vi "reward_behavior_michelle_visjitter_conswinAdapt_enticefx_TSLog_VF_withvid.vi"() -> ()   [LabVIEW 2019]
doc: "The myRIO Project template acquires acceleration data from the onboard accelerometer and displays the changes of acceleration values in a waveform chart."
uses:
  <vilib>/Analysis/Matrix/Datatypes/RealMatrix.ctl
  <vilib>/myRIO/Instrument Drivers/Onboard IO/DIO/typedefs/DIO Reference.ctl
  <vilib>/myRIO/Common/Instrument Driver Framework/Utilities/typedefs/myRIO Generic Hardware Reference.ctl
  <vilib>/myRIO/Common/Instrument Driver Framework/Utilities/typedefs/Hardware Version Enum.ctl
  <vilib>/myRIO/Common/Instrument Driver Framework/Utilities/typedefs/myRIO v1.0 Reference.ctl
  <vilib>/myRIO/Common/Instrument Driver Framework/Utilities/typedefs/Generic FPGA Reference.ctl
  <vilib>/myRIO/Common/Instrument Driver Framework/myRIO v1.0/DIO/typedefs/DIO Channels List.ctl
  <vilib>/myRIO/Common/Instrument Driver Framework/myRIO v1.0/DIO/typedefs/DIO Channels Enum.ctl
  <vilib>/userdefined/High Color/nirio_resource_hc.ctl
  <vilib>/myRIO/Common/Instrument Driver Framework/myRIO v1.0/Encoder/typedefs/Encoder Signal Mode.ctl
  <vilib>/myRIO/Instrument Drivers/Onboard IO/Encoder/typedefs/Encoder Reference.ctl
  <vilib>/myRIO/Common/Instrument Driver Framework/myRIO v1.0/Encoder/typedefs/Encoder Channels Enum.ctl
  <vilib>/myRIO/Common/Instrument Driver Framework/myRIO v1.0/Encoder/typedefs/Encoder Configuration v1.0.ctl
  <vilib>/myRIO/Common/Instrument Driver Framework/Utilities/vis/Is FPGA Ref Available.vi
  <vilib>/myRIO/Common/Instrument Driver Framework/myRIO v1.0/DIO/vis/myRIO v1.1 Open DIO.vi
  <vilib>/myRIO/Instrument Drivers/Onboard IO/DIO/vis/Write.vi
  <vilib>/myRIO/Common/Instrument Driver Framework/myRIO v1.0/Encoder/vis/myRIO v1.1 Open Encoder.vi
  <vilib>/myRIO/Instrument Drivers/Onboard IO/Encoder/vis/Read.vi
  <vilib>/myRIO/Instrument Drivers/Onboard IO/DIO/vis/Read.vi
  <vilib>/myRIO/Common/Instrument Driver Framework/Utilities/vis/Validate Channels.vi
  <vilib>/myRIO/Common/Instrument Driver Framework/myRIO v1.0/DIO/vis/myRIO v1.0 Reserve DIO.vi
  <vilib>/myRIO/Common/Instrument Driver Framework/myRIO v1.0/Encoder/vis/myRIO v1.0 Reserve Encoder.vi
  <vilib>/myRIO/Common/Instrument Driver Framework/myRIO v1.0/Resource Manager/vis/myRIO v1.0 Reserve Channel List.vi
  <vilib>/myRIO/Common/Instrument Driver Framework/myRIO v1.0/DIO/vis/myRIO v1.0 Build MUX Configuration DIO.vi
  <vilib>/myRIO/Common/Instrument Driver Framework/myRIO v1.0/Encoder/vis/myRIO v1.0 Build MUX Configuration Encoder.vi
  <vilib>/myRIO/Common/Instrument Driver Framework/myRIO v1.0/Resource Manager/vis/myRIO v1.0 Reserve Channel.vi
  <vilib>/myRIO/Common/Instrument Driver Framework/myRIO v1.0/Resource Manager/vis/myRIO v1.0 Unreserve Channel.vi
  <vilib>/myRIO/Common/Instrument Driver Framework/myRIO v1.0/Resource Manager/vis/myRIO v1.0 Create Configuration List.vi
  <vilib>/myRIO/Common/Instrument Driver Framework/myRIO v1.0/Resource Manager/vis/myRIO v1.0 Build Mutex Name.vi
  <vilib>/Utility/VariantDataType/GetNumericInfo.vi
  <vilib>/Utility/error.llb/Error Cluster From Error Code.vi
  <vilib>/myRIO/Common/Instrument Driver Framework/myRIO v1.0/myRIO v1.1 Open.vi
  <vilib>/myRIO/Common/Instrument Driver Framework/Utilities/vis/IO Manager.vi
  <vilib>/myRIO/Common/Instrument Driver Framework/Utilities/vis/Configuration Manager.vi
  <vilib>/myRIO/Common/Instrument Driver Framework/myRIO v1.0/Resource Manager/vis/myRIO v1.0 Configure IO.vi
  <vilib>/myRIO/Common/Instrument Driver Framework/myRIO v1.0/myRIO v1.0 Close.vi
  <vilib>/myRIO/Common/Instrument Driver Framework/myRIO v1.0/Encoder/vis/myRIO v1.0 Configure Encoder.vi
  <vilib>/myRIO/Common/Instrument Driver Framework/myRIO v1.0/Encoder/vis/myRIO v1.0 Read Encoder.vi
  <vilib>/myRIO/Common/Instrument Driver Framework/myRIO v1.0/DIO/vis/myRIO v1.0 Write DIO.vi
  <vilib>/myRIO/Common/Instrument Driver Framework/myRIO v1.0/DIO/vis/myRIO v1.0 Read DIO.vi
  <vilib>/myRIO/Express VI/Onboard IO/Encoder/Encoder Express VI.xnode
  <vilib>/myRIO/Instrument Drivers/Onboard IO/Encoder/vis/myRIO Encoder Open.xnode
  <vilib>/myRIO/Common/Instrument Driver Framework/myRIO v1.0/Encoder/typedefs/Encoder Count Direction Enum.ctl
  <vilib>/myRIO/Express VI/Onboard IO/DO/DO Express VI.xnode
  <vilib>/myRIO/Instrument Drivers/Onboard IO/DIO/vis/myRIO DIO Open.xnode
  <vilib>/myRIO/Express VI/Onboard IO/DI/DI Express VI.xnode
  <vilib>/myRIO/Instrument Drivers/Onboard IO/Encoder/Encoder.lvlib
  <vilib>/myRIO/Instrument Drivers/Onboard IO/DIO/DIO.lvlib
  <vilib>/Analysis/Matrix/NI_Matrix.lvlib
panel:
  out "GetVidFrame":i32
  out "VidTS":dbl[][](array[numeric])
  out "VidFrameClock":i32
  out "EntTS":dbl[][](array[numeric])
  out "TimeLag":dbl
  out "Lag2":dbl
  out "TestTime":dbl
  out "RewTS":dbl[][](array[numeric])
  out "ConsTS":dbl[][](array[numeric])
  out "LickTS":dbl[][](array[numeric])
  out "ContrastChoice":dbl
  out "Its":i32
  out "BurstCriteria":dbl
  out "LickBurst 2":bool
  out "LickBurst":bool
  out "Enticements":i32
  in  "Entice":bool
  out "Misses":i32
  out "GoAhead":bool
  out "TimeOutDuration":i32
  out "ActiveTime":dbl
  out "ConsumptionGo":bool=TRUE
  out "Consumption_Period":i32
  out "Watch_Display":bool=TRUE
  in  "Give reward":bool
  out "Timings":dbl[](array[numeric])
  out "ISI":dbl
  out "ISI start time":dbl
  out "Time_out":bool=TRUE
  out "Time since lick":dbl
  out "Time of last lick":dbl
  out "Rewarded trials":dbl[](array[numeric])
  out "Rewards":u16
  out "Active Trial":bool
  out "Array temp2":T1
  out "Stimuli Loaded":bool
  out "Stim_ID":dbl[](array[numeric])
  out "Reward_mat":dbl[](array[numeric])
  out "Reward":bool=TRUE
  out "Frame clock":i32
  out "Licks":u32
  out "Lick":bool
  out "Time":dbl
  out "Stop":bool
  in  "Frames to collect":u32
  out "Overflow?":bool
  out "Counter Value":i32
  out "Velocity":dbl
  out "Velocity Plot":dbl[](graph)
  out "Velocity array":dbl[](array[numeric])
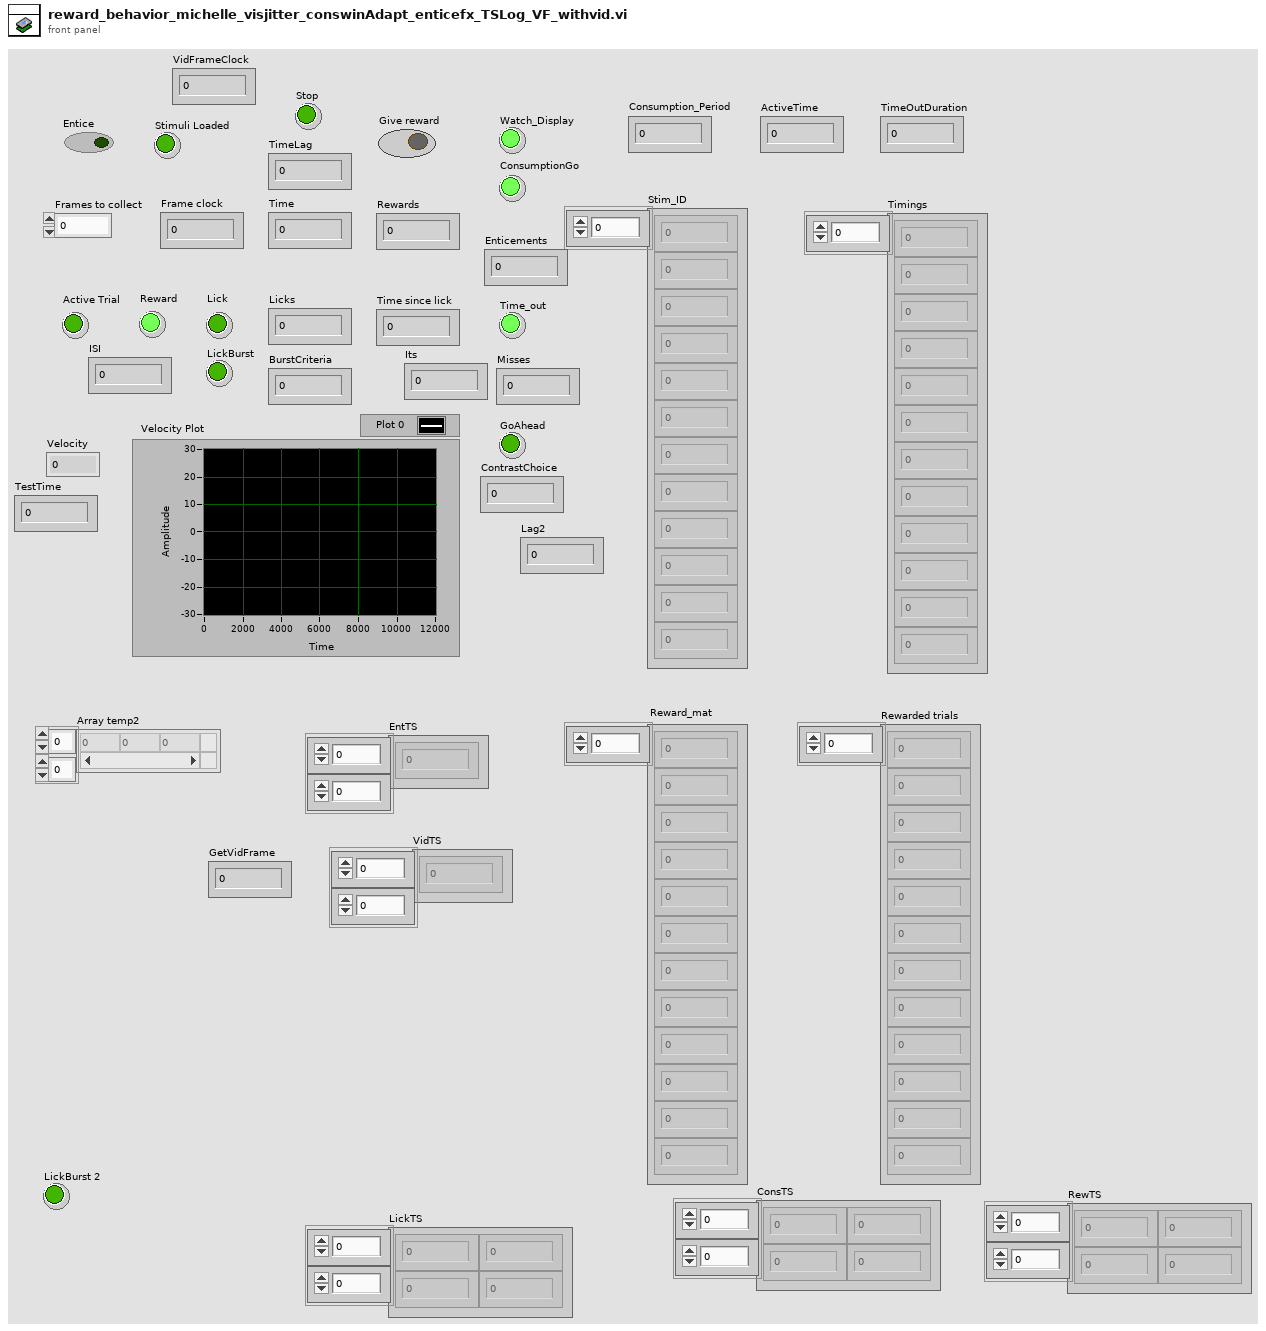
[diagram p1: front panel]
types:
  T1 = typedef "NI_Matrix.lvlib/RealMatrix.ctl" = dbl[][]
  T2 = typedef "DIO.lvlib/DIO Reference.ctl" = cluster{"myRIO Reference":T3, "DIO Channels List":T7}
  T3 = typedef "myRIO Generic Hardware Reference.ctl" = cluster{"myRIO Model":T4, "myRIO Hardware Reference":T5}
  T4 = typedef "Hardware Version Enum.ctl" = enum16{"Unknown", "myRIO-1900", "myRIO-1950", "roboRIO", "NI ELVIS RIO CM", "ELVIS III"}
  T5 = typedef "myRIO v1.0 Reference.ctl" = cluster{"Generic FPGA Reference":T6, "Allow multiple opens":bool}
  T6 = typedef "Generic FPGA Reference.ctl" = refnum<k20>
  T7 = typedef "DIO Channels List.ctl" = T8[]
  T8 = typedef "DIO Channels Enum.ctl" = enum16{"Not Connected", "C/DIO0", "C/DIO1", "C/DIO2", "C/DIO3", "C/DIO4", "C/DIO5", "C/DIO6", "C/DIO7", "A/DIO0", "A/DIO1", "A/DIO2", "A/DIO3", "A/DIO4", "A/DIO5", "A/DIO6", "A/DIO7", "A/DIO8", "A/DIO9", "A/DIO10", "A/DIO11", "A/DIO12", "A/DIO13", "A/DIO14", "A/DIO15", "A/DIO16", "A/DIO17", "A/DIO18", "A/DIO19", "B/DIO0", "B/DIO1", "B/DIO2", "B/DIO3", "B/DIO4", "B/DIO5", "B/DIO6", "B/DIO7", "B/DIO8", "B/DIO9", "B/DIO10", "B/DIO11", "B/DIO12", "B/DIO13", "B/DIO14", "B/DIO15", "B/DIO16", "B/DIO17", "B/DIO18", "B/DIO19", "LED0", "LED1", "LED2", "LED3", "Button0", "DIO/DIO0", "DIO/DIO1", "DIO/DIO2", "DIO/DIO3", "DIO/DIO4", "DIO/DIO5", "DIO/DIO6", "DIO/DIO7", "DIO/DIO8", "DIO/DIO9", "SPI/CS0", "SPI/CS1", "SPI/CS2", "SPI/CS3", "LED RADIO (Green)", "LED RADIO (Red)", "LED COMM (Green)", "LED COMM (Red)", "LED MODE (Green)", "LED MODE (Red)"}
  T9 = typedef "nirio_resource_hc.ctl" = tag
  T10 = typedef "Encoder.lvlib/Encoder Reference.ctl" = cluster{"myRIO Reference":T3, "Encoder Channels Enum":T11}
  T11 = typedef "Encoder Channels Enum.ctl" = enum16{"Not Connected", "C/ENC0", "C/ENC1", "A/ENC", "A/ENC0", "A/ENC1", "A/ENC2", "A/ENC3", "A/ENC4", "A/ENC5", "A/ENC6", "A/ENC7", "A/ENC8", "A/ENC9", "B/ENC", "B/ENC0", "B/ENC1", "B/ENC2", "B/ENC3", "B/ENC4", "B/ENC5", "B/ENC6", "B/ENC7", "B/ENC8", "B/ENC9", "DIO/ENC0", "DIO/ENC1", "DIO/ENC2", "DIO/ENC3", "DIO/ENC4"}
  T12 = typedef "Encoder Signal Mode.ctl" = enum16{"Quadrature phase signal", "Step and direction signal"}
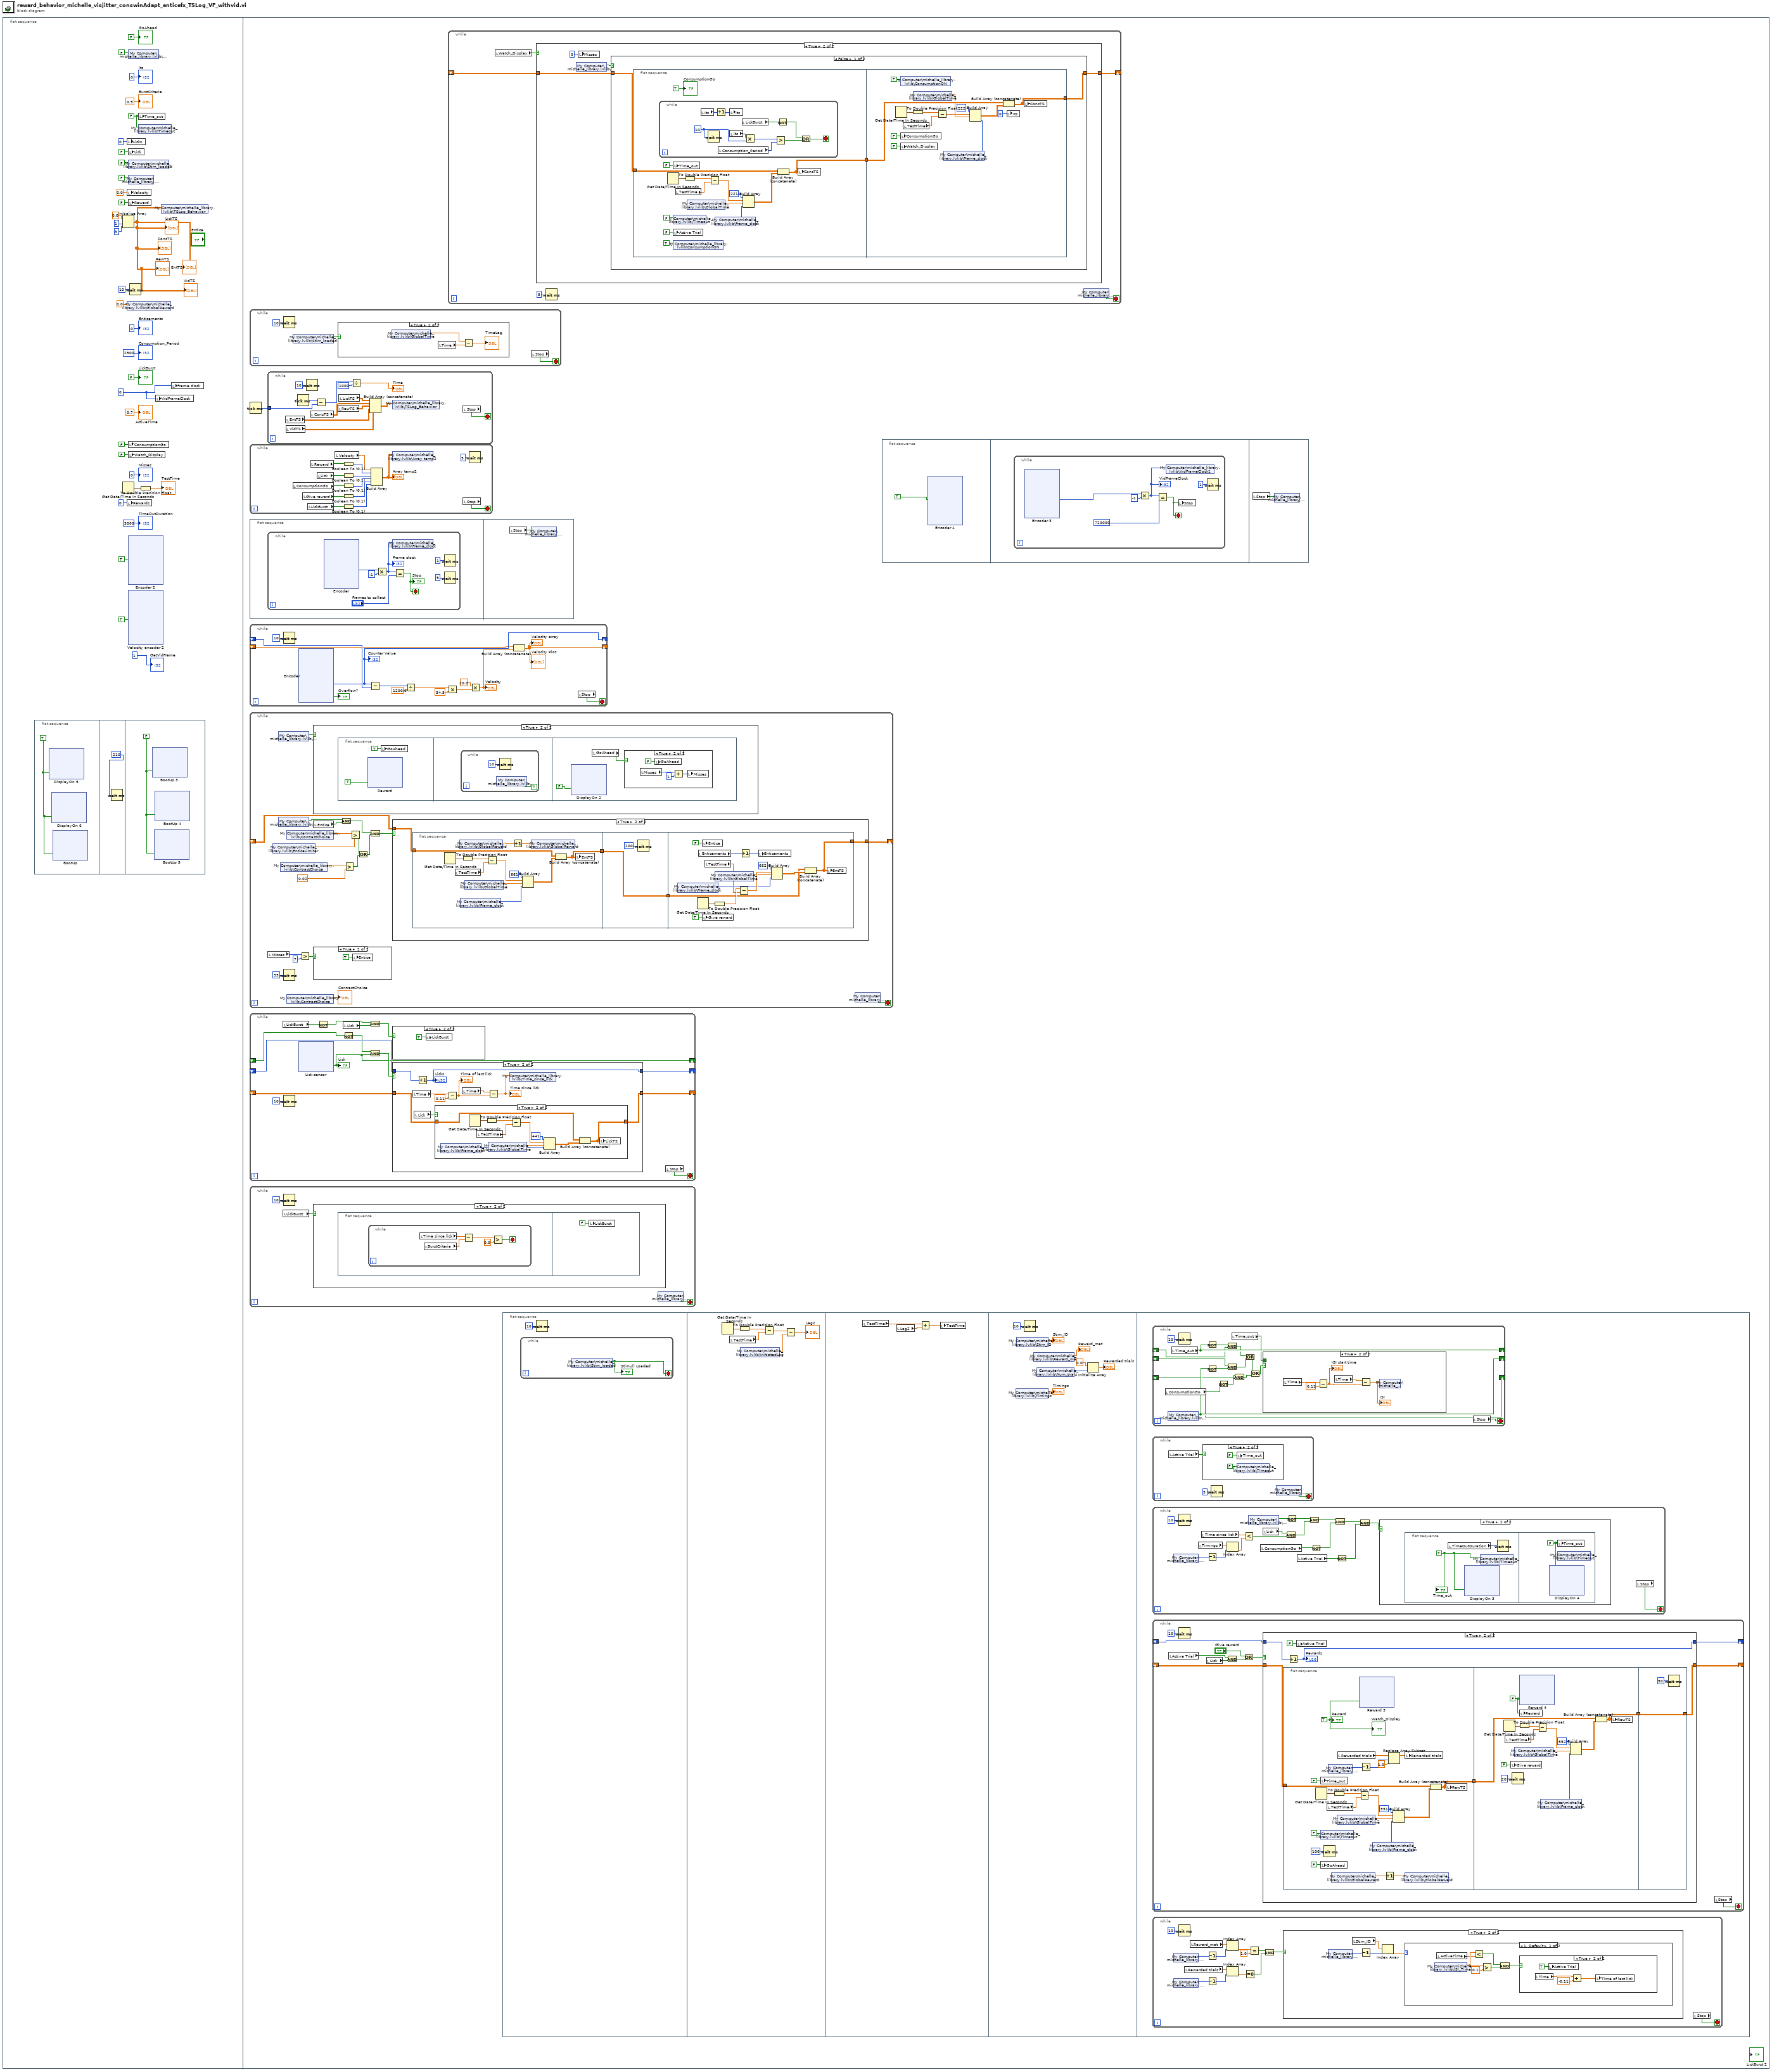
[diagram p0: block diagram]
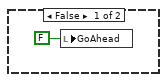
[diagram p6: hidden frame]
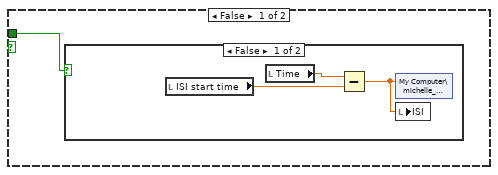
[diagram p12: hidden frame]
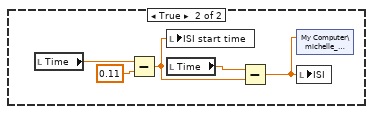
[diagram p13: hidden frame]
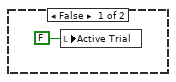
[diagram p14: hidden frame]
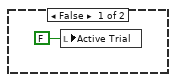
[diagram p15: hidden frame]
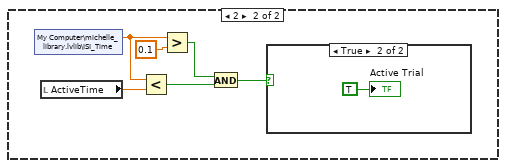
[diagram p16: hidden frame]
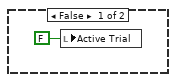
[diagram p17: hidden frame]
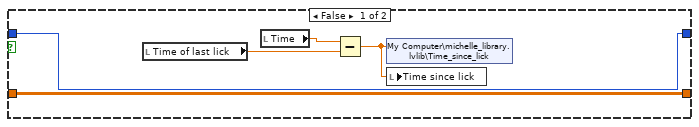
[diagram p20: hidden frame]
diagram:
  n1 = flat-sequence {
    frame #0 {
      w21 = FALSE ("Time_out")
      w3 = u32 0 ("Frames")
      n2 = flat-sequence {
        frame #0 {
          w33 = TRUE
          n3 = xnode "DisplayOn 5"("C/DIO2 (DIO2)"=w33) -> ()  [unwired: 1 in, 1 out]
          n4 = xnode "DisplayOn 6"("C/DIO1 (DIO1)"=w33) -> ()  [unwired: 1 in, 1 out]
          n5 = xnode "BootUp"("C/DIO3 (DIO3)"=w33) -> ()  [unwired: 1 in, 1 out]
        }
        frame #1 {
          n6 = Wait (ms)(milliseconds to wait=210) -> ()  [unwired: 1 out]
        }
        frame #2 {
          w140 = FALSE
          n7 = xnode "BootUp 3"("C/DIO2 (DIO2)"=w140) -> ()  [unwired: 1 in, 1 out]
          n8 = xnode "BootUp 5"("C/DIO3 (DIO3)"=w140) -> ()  [unwired: 1 in, 1 out]
          n9 = xnode "BootUp 4"("C/DIO1 (DIO1)"=w140) -> ()  [unwired: 1 in, 1 out]
        }
      }
      n10 = Get Date/Time In Seconds() -> (seconds since 1Jan1904=w5:timestamp)
      n11 = Initialize Array(0.0, 1, 3) -> (w2:dbl[][])
      "LickTS" <- w2
      "ConsTS" <- w2
      "RewTS" <- w2
      "EntTS" <- w2
      "VidTS" <- w2
      n12 = local write "Licks"(u32 0 ("Licks")) -> ()
      n13 = local write "Velocity"(0.0 ("Velocity")) -> ()
      n14 = shared-variable "My Computer\\michelle_library.lvlib\\GlobalReward"(0.0) -> ()  [unwired: 1 in, 1 out]
      n15 = local write "Rewards"(u16 0 ("Rewards")) -> ()
      n16 = shared-variable "My Computer\\michelle_library.lvlib\\Display"(FALSE ("Display")) -> ()  [unwired: 1 in, 1 out]
      n17 = local write "Lick"(FALSE ("Lick")) -> ()
      n18 = shared-variable "My Computer\\michelle_library.lvlib\\Stim_loaded"(FALSE ("Stim_loaded")) -> ()  [unwired: 1 in, 1 out]
      n19 = shared-variable "My Computer\\michelle_library.lvlib\\Stop"(FALSE ("Stop")) -> ()  [unwired: 1 in, 1 out]
      n20 = local write "Reward"(FALSE ("Give reward")) -> ()
      n21 = local write "ConsumptionGo"(FALSE ("ConsumptionGo")) -> ()
      n22 = local write "Watch_Display"(FALSE ("Watch_Display")) -> ()
      n23 = xnode "Encoder 2"("Reset Counter"=TRUE) -> ()  [unwired: 1 in, 4 out]
      n24 = xnode "Velocity encoder 2"("Reset Counter"=TRUE) -> ()  [unwired: 1 in, 4 out]
      n25 = Wait (ms)(milliseconds to wait=u32 10) -> ()  [unwired: 1 out]
      n26 = local write "Time_out"(w21) -> ()
      n27 = shared-variable "My Computer\\michelle_library.lvlib\\Timeout"(w21) -> ()  [unwired: 1 in, 1 out]
      n28 = To Double Precision Float(number=w5) -> (double precision float=→"TestTime":dbl)
      n29 = local write "VidFrameClock"(w3) -> ()
      n30 = shared-variable "My Computer\\michelle_library.lvlib\\TSLog_Behavior"(w2) -> ()  [unwired: 1 in, 1 out]
      n31 = local write "Frame clock"(w3) -> ()
      "Consumption_Period" <- 2500
      "ActiveTime" <- 0.7
      "TimeOutDuration" <- 3000
      "GoAhead" <- FALSE
      "Misses" <- 0
      "Enticements" <- 0
      "LickBurst" <- FALSE
      "BurstCriteria" <- 0.5
      "Its" <- 0
      "GetVidFrame" <- 1
    }
    frame #1 {
      n32 = while {
        stop <- w440 stop-if-true
        n33 = Wait (ms)(milliseconds to wait=u32 10) -> ()  [unwired: 1 out]
        n34 = shared-variable "My Computer\\michelle_library.lvlib\\Stim_loaded"() -> (w441:bool)  [unwired: 1 in, 1 out]
        n35 = case shown="True" w441 {
          frame False {
          }
          frame True {
            n36 = shared-variable "My Computer\\michelle_library.lvlib\\GlobalTime"() -> (w442:dbl)  [unwired: 1 in, 1 out]
            n37 = local read "Time"() -> (w443:dbl)
            n38 = Subtract(x=w442, y=w443) -> (x-y=→"TimeLag":dbl)
          }
        }
        n39 = local read "Stop"() -> (w440:bool)
      }
      n40 = Tick Count (ms)() -> (millisecond timer value=w338:u32)
      n41 = while {
        stop <- w649 stop-if-true
        n42 = local read "ConsumptionGo"() -> (w647:bool)
        n43 = local read "Give reward"() -> (w646:bool)
        n44 = local read "LickBurst"() -> (w643:bool)
        n45 = local read "Reward"() -> (w654:bool)
        n46 = local read "Lick"() -> (w655:bool)
        n47 = local read "Velocity"() -> (w653:dbl)
        n48 = Boolean To (0,1)(Boolean=w654) -> (0, 1=w652:i16)
        n49 = Boolean To (0,1)(Boolean=w655) -> (0, 1=w651:i16)
        n50 = Boolean To (0,1)(Boolean=w647) -> (0, 1=w645:i16)
        n51 = Boolean To (0,1)(Boolean=w646) -> (0, 1=w644:i16)
        n52 = Boolean To (0,1)(Boolean=w643) -> (0, 1=w642:i16)
        n53 = Build Array(w653, w652, w651, w645, w644, w642) -> (w648:T1)
        "Array temp2" <- w648
        n54 = shared-variable "My Computer\\michelle_library.lvlib\\Array temp2"(w648) -> ()  [unwired: 1 in, 1 out]
        n55 = local read "Stop"() -> (w649:bool)
        n56 = Wait (ms)(milliseconds to wait=u32 5) -> ()  [unwired: 1 out]
      }
      n57 = flat-sequence {
        frame #0 {
          n58 = while {
            stop <- w968 stop-if-true
            n59 = xnode "Encoder"() -> ("Counter Value"=w972:i32)  [unwired: 2 in, 3 out]
            n60 = Multiply(x=w972, y=-1) -> (x*y=w967:i32)
            "Frame clock" <- w967
            n61 = shared-variable "My Computer\\michelle_library.lvlib\\Frame_clock"(w967) -> ()  [unwired: 1 in, 1 out]
            n62 = Equal?(x=w967, y="Frames to collect") -> (x = y?=w968:bool)
            "Stop" <- w968
            n63 = Wait (ms)(milliseconds to wait=u32 1) -> ()  [unwired: 1 out]
            n64 = Wait (ms)(milliseconds to wait=u32 5) -> ()  [unwired: 1 out]
          }
        }
        frame #1 {
          n65 = local read "Stop"() -> (w1020:bool)
          n66 = shared-variable "My Computer\\michelle_library.lvlib\\Stop"(w1020) -> ()  [unwired: 1 in, 1 out]
        }
      }
      n67 = while {
        shift-right: [w1107] -> _
        shift-left: _ -> [w1108]
        shift-right: [w1099] -> _
        shift-left: _ -> [w1098]
        stop <- w1097 stop-if-true
        n68 = Wait (ms)(milliseconds to wait=u32 10) -> ()  [unwired: 1 out]
        n69 = xnode "Encoder"() -> ("Counter Value"=w1107:i32, "Overflow?"=→"Overflow?":bool)  [unwired: 2 in, 2 out]
        "Counter Value" <- w1107
        n70 = Subtract(x=w1107, y=w1108) -> (x-y=w1100:i32)
        n71 = Divide(x=w1100, y=1200.0 ("600")) -> (x/y=w1105:dbl)
        n72 = Multiply(x=w1105, y=34.5) -> (x*y=w1103:dbl)
        n73 = Multiply(x=20.0, y=w1103) -> (x*y=w1101:dbl)
        "Velocity" <- w1101
        n74 = Build Array (concatenate)(w1098, w1101) -> (w1099:dbl[])
        "Velocity Plot" <- w1099
        "Velocity array" <- w1099
        n75 = local read "Stop"() -> (w1097:bool)
      }
      n76 = while {
        shift-right: [w460] -> _
        shift-left: _ -> [w461]
        stop <- w473 stop-if-true
        n77 = local read "Misses"() -> (w471:i32)
        n78 = shared-variable "My Computer\\michelle_library.lvlib\\EnticeLimiter"() -> (w459:dbl)  [unwired: 1 in, 1 out]
        n79 = shared-variable "My Computer\\michelle_library.lvlib\\Display"() -> (w472:bool)  [unwired: 1 in, 1 out]
        n80 = shared-variable "My Computer\\michelle_library.lvlib\\Display"() -> (w468:bool)  [unwired: 1 in, 1 out]
        n81 = shared-variable "My Computer\\michelle_library.lvlib\\ContrastChoice"() -> (w455:dbl)  [unwired: 1 in, 1 out]
        n82 = Wait (ms)(milliseconds to wait=35) -> ()  [unwired: 1 out]
        n83 = shared-variable "My Computer\\michelle_library.lvlib\\ContrastChoice"() -> (w464:dbl)  [unwired: 1 in, 1 out]
        n84 = shared-variable "My Computer\\michelle_library.lvlib\\ContrastChoice"() -> (→"ContrastChoice":dbl)  [unwired: 1 in, 1 out]
        n85 = Greater?(x=w471, y=7) -> (0:w469:bool)
        n86 = case shown="True" w472 {
          frame False {
            n87 = local write "GoAhead"(FALSE) -> ()
          }
          frame True {
            n88 = flat-sequence {
              frame #0 {
                n89 = xnode "Reward"("C/DIO2 (DIO2)"=TRUE) -> ()  [unwired: 1 in, 1 out]
                n90 = local write "GoAhead"(TRUE) -> ()
              }
              frame #1 {
                n91 = while {
                  stop <- w547 continue-if-true
                  n92 = shared-variable "My Computer\\michelle_library.lvlib\\Display"() -> (w547:bool)  [unwired: 1 in, 1 out]
                  n93 = Wait (ms)(milliseconds to wait=10) -> ()  [unwired: 1 out]
                }
              }
              frame #2 {
                n94 = xnode "DisplayOn 2"("C/DIO2 (DIO2)"=FALSE) -> ()  [unwired: 1 in, 1 out]
                n95 = local read "GoAhead"() -> (w549:bool)
                n96 = case shown="True" w549 {
                  frame False {
                  }
                  frame True {
                    n97 = local read "Misses"() -> (w588:i32)
                    n98 = local write "GoAhead"(FALSE) -> ()
                    n99 = Add(x=w588, y=1) -> (x+y=w586:i32)
                    n100 = local write "Misses"(w586) -> ()
                  }
                }
              }
            }
          }
        }
        n101 = local read "Entice"() -> (w467:bool)
        n102 = case shown="True" w469 {
          frame False {
          }
          frame True {
            n103 = local write "Entice"(TRUE) -> ()
          }
        }
        n104 = And(x=w468, y=w467) -> (x .and. y?=w465:bool)
        n105 = Greater?(x=w455, y=0.02) -> (0:w456:bool)
        n106 = Greater?(x=w464, y=w459) -> (0:w457:bool)
        n107 = Or(x=w457, y=w456) -> (x .or. y?=w458:bool)
        n108 = And(x=w465, y=w458) -> (x .and. y?=w463:bool)
        n109 = case shown="True" w463 {
          tunnel: w461 -> [w474 w478]
          tunnel: [w474 w475] -> w460
          frame False {
          }
          frame True {
            n110 = flat-sequence {
              tunnel: w478 -> [w481]
              tunnel: [w480] -> w477
              tunnel: w477 -> [w491]
              tunnel: [w491] -> w476
              tunnel: w476 -> [w495]
              tunnel: [w494] -> w475
              frame #0 {
                n111 = Get Date/Time In Seconds() -> (seconds since 1Jan1904=w488:timestamp)
                n112 = local read "TestTime"() -> (w483:dbl)
                n113 = shared-variable "My Computer\\michelle_library.lvlib\\GlobalReward"() -> (w490:dbl)  [unwired: 1 in, 1 out]
                n114 = shared-variable "My Computer\\michelle_library.lvlib\\Frame_clock"() -> (w479:u32)  [unwired: 1 in, 1 out]
                n115 = To Double Precision Float(number=w488) -> (double precision float=w487:dbl)
                n116 = shared-variable "My Computer\\michelle_library.lvlib\\GlobalTime"() -> (w482:dbl)  [unwired: 1 in, 1 out]
                n117 = Subtract(x=w487, y=w483) -> (x-y=w486:dbl)
                n118 = Increment(x=w490) -> (x+1=w489:dbl)
                n119 = Build Array(661, w486, w482, w479) -> (w485:T1)
                n120 = shared-variable "My Computer\\michelle_library.lvlib\\GlobalReward"(w489) -> ()  [unwired: 1 in, 1 out]
                n121 = Build Array (concatenate) ("Build Matrix")(w481, w485) -> (w480:T1)
                n122 = local write "EntTS"(w480) -> ()
              }
              frame #1 {
                n123 = Wait (ms)(milliseconds to wait=200) -> ()  [unwired: 1 out]
              }
              frame #2 {
                n124 = shared-variable "My Computer\\michelle_library.lvlib\\Frame_clock"() -> (w493:u32)  [unwired: 1 in, 1 out]
                n125 = Get Date/Time In Seconds() -> (seconds since 1Jan1904=w502:timestamp)
                n126 = local read "Enticements"() -> (w504:i32)
                n127 = local write "Entice"(FALSE) -> ()
                n128 = local write "Give reward"(TRUE) -> ()
                n129 = local read "TestTime"() -> (w496:dbl)
                n130 = To Double Precision Float(number=w502) -> (double precision float=w501:dbl)
                n131 = shared-variable "My Computer\\michelle_library.lvlib\\GlobalTime"() -> (w497:dbl)  [unwired: 1 in, 1 out]
                n132 = Subtract(x=w501, y=w496) -> (x-y=w500:dbl)
                n133 = Increment(x=w504) -> (x+1=w503:i32)
                n134 = local write "Enticements"(w503) -> ()
                n135 = Build Array(662, w500, w497, w493) -> (w499:T1)
                n136 = Build Array (concatenate) ("Build Matrix")(w495, w499) -> (w494:T1)
                n137 = local write "EntTS"(w494) -> ()
              }
            }
          }
        }
        n138 = shared-variable "My Computer\\michelle_library.lvlib\\Stop"() -> (w473:bool)  [unwired: 1 in, 1 out]
      }
      n139 = while {
        shift-right: [w1033] -> _
        shift-left: _ -> [w1032]
        shift-right: [w1027] -> _
        shift-left: _ -> [w1030]
        shift-right: [w1021] -> _
        shift-left: _ -> [w1022]
        stop <- w1031 stop-if-true
        n140 = local read "LickBurst"() -> (w1024:bool)
        n141 = Wait (ms)(milliseconds to wait=u32 10) -> ()  [unwired: 1 out]
        n142 = xnode "Lick sensor"() -> ("C/DIO1 (DIO1)"=w1027:bool)  [unwired: 1 in, 1 out]
        "Lick" <- w1027
        n143 = Not(x=w1024) -> (.not. x?=w1023:bool)
        n144 = Not(x=w1030) -> (.not. x?=w1029:bool)
        n145 = local read "Lick"() -> (w1025:bool)
        n146 = And(x=w1023, y=w1025) -> (x .and. y?=w1026:bool)
        n147 = And(x=w1029, y=w1027) -> (x .and. y?=w1028:bool)
        n148 = case shown="True" w1026 {
          frame False {
          }
          frame True {
            n149 = local write "LickBurst"(TRUE) -> ()
          }
        }
        n150 = case shown="True" w1028 {
          tunnel: [w1040 w1050] -> w1033
          tunnel: w1032 -> [w1040 w1049]
          tunnel: w1022 -> [w1036 w1041]
          tunnel: [w1036 w1043] -> w1021
          frame False {
            n151 = local read "Time of last lick"() -> (w1038:dbl)
            n152 = local read "Time"() -> (w1039:dbl)
            n153 = Subtract(x=w1039, y=w1038) -> (x-y=w1037:dbl)
            n154 = shared-variable "My Computer\\michelle_library.lvlib\\Time_since_lick"(w1037) -> ()  [unwired: 1 in, 1 out]
            n155 = local write "Time since lick"(w1037) -> ()
          }
          frame True {
            n156 = local read "Time"() -> (w1046:dbl)
            n157 = local read "Lick"() -> (w1042:bool)
            n158 = Increment(x=w1049) -> (x+1=w1050:u32)
            "Licks" <- w1050
            n159 = case shown="True" w1042 {
              tunnel: w1041 -> [w1051 w1057]
              tunnel: [w1051 w1056] -> w1043
              frame False {
              }
              frame True {
                n160 = shared-variable "My Computer\\michelle_library.lvlib\\Frame_clock"() -> (w1052:u32)  [unwired: 1 in, 1 out]
                n161 = Get Date/Time In Seconds() -> (seconds since 1Jan1904=w1059:timestamp)
                n162 = local read "TestTime"() -> (w1054:dbl)
                n163 = To Double Precision Float(number=w1059) -> (double precision float=w1055:dbl)
                n164 = shared-variable "My Computer\\michelle_library.lvlib\\GlobalTime"() -> (w1053:dbl)  [unwired: 1 in, 1 out]
                n165 = Subtract(x=w1055, y=w1054) -> (x-y=w1060:dbl)
                n166 = Build Array(441, w1060, w1053, w1052) -> (w1061:T1)
                n167 = Build Array (concatenate) ("Build Matrix")(w1057, w1061) -> (w1056:T1)
                n168 = local write "LickTS"(w1056) -> ()
              }
            }
            n169 = Subtract(x=w1046, y=0.11) -> (x-y=w1044:dbl)
            "Time of last lick" <- w1044
            n170 = local read "Time"() -> (w1048:dbl)
            n171 = Subtract(x=w1048, y=w1044) -> (x-y=w1047:dbl)
            "Time since lick" <- w1047
            n172 = shared-variable "My Computer\\michelle_library.lvlib\\Time_since_lick"(w1047) -> ()  [unwired: 1 in, 1 out]
          }
        }
        n173 = local read "Stop"() -> (w1031:bool)
      }
      n174 = while {
        stop <- w447 stop-if-true
        n175 = local read "LickBurst"() -> (w445:bool)
        n176 = Wait (ms)(milliseconds to wait=u32 10) -> ()  [unwired: 1 out]
        n177 = case shown="True" w445 {
          frame False {
          }
          frame True {
            n178 = flat-sequence {
              frame #0 {
                n179 = while {
                  stop <- w450 stop-if-true
                  n180 = local read "Time since lick"() -> (w451:dbl)
                  n181 = local read "BurstCriteria"() -> (w452:dbl)
                  n182 = Subtract(x=w451, y=w452) -> (x-y=w448:dbl)
                  n183 = Greater?(x=w448, y=0.0) -> (0:w450:bool)
                }
              }
              frame #1 {
                n184 = local write "LickBurst"(FALSE) -> ()
              }
            }
          }
        }
        n185 = shared-variable "My Computer\\michelle_library.lvlib\\Stop"() -> (w447:bool)  [unwired: 1 in, 1 out]
      }
      n186 = while {
        tunnel: w338 -> [w1168]
        stop <- w1166 stop-if-true
        n187 = local read "EntTS"() -> (w1158:dbl[][])
        n188 = local read "VidTS"() -> (w1157:dbl[][])
        n189 = Tick Count (ms)() -> (millisecond timer value=w1169:u32)
        n190 = Wait (ms)(milliseconds to wait=u32 10) -> ()  [unwired: 1 out]
        n191 = local read "ConsTS"() -> (w1161:dbl[][])
        n192 = Subtract(x=w1169, y=w1168) -> (x-y=w1165:u32)
        n193 = local read "RewTS"() -> (w1160:dbl[][])
        n194 = local read "LickTS"() -> (w1162:dbl[][])
        n195 = Divide(x=w1165, y=u32 1000) -> (x/y=→"Time":dbl)
        n196 = Build Array (concatenate) ("Build Matrix")(w1162, w1161, w1160, w1158, w1157) -> (w1159:T1)
        n197 = shared-variable "My Computer\\michelle_library.lvlib\\TSLog_Behavior"(w1159) -> ()  [unwired: 1 in, 1 out]
        n198 = local read "Stop"() -> (w1166:bool)
      }
      n199 = while {
        shift-right: [w589] -> _
        shift-left: _ -> [w590]
        stop <- w593 stop-if-true
        n200 = local read "Watch_Display"() -> (w592:bool)
        n201 = case shown="True" w592 {
          tunnel: w590 -> [w594 w596]
          tunnel: [w594 w595] -> w589
          frame False {
          }
          frame True {
            n202 = shared-variable "My Computer\\michelle_library.lvlib\\Display"() -> (w598:bool)  [unwired: 1 in, 1 out]
            n203 = local write "Misses"(0) -> ()
            n204 = case shown="False" w598 {
              tunnel: w596 -> [w601 w641]
              tunnel: [w599 w641] -> w595
              frame False {
                n205 = flat-sequence {
                  tunnel: w601 -> [w605]
                  tunnel: [w604] -> w600
                  tunnel: w600 -> [w631]
                  tunnel: [w630] -> w599
                  frame #0 {
                    n206 = while {
                      stop <- w620 stop-if-true
                      w621 = 10
                      n207 = local read "Its"() -> (w625:i32)
                      n208 = Wait (ms)(milliseconds to wait=w621) -> ()  [unwired: 1 out]
                      n209 = Increment(x=w625) -> (x+1=w624:i32)
                      n210 = local read "Consumption_Period"() -> (w618:i32)
                      n211 = local write "Its"(w624) -> ()
                      n212 = local read "Its"() -> (w622:i32)
                      n213 = local read "LickBurst"() -> (w626:bool)
                      n214 = Multiply(x=w622, y=w621) -> (x*y=w619:i32)
                      n215 = Greater?(x=w619, y=w618) -> (0:w617:bool)
                      n216 = Not(x=w626) -> (.not. x?=w623:bool)
                      n217 = Or(x=w623, y=w617) -> (x .or. y?=w620:bool)
                    }
                    n218 = Get Date/Time In Seconds() -> (seconds since 1Jan1904=w610:timestamp)
                    n219 = local write "Time_out"(FALSE) -> ()
                    n220 = shared-variable "My Computer\\michelle_library.lvlib\\Timeout"(FALSE) -> ()  [unwired: 1 in, 1 out]
                    n221 = local write "Active Trial"(FALSE) -> ()
                    n222 = shared-variable "My Computer\\michelle_library.lvlib\\ConsumptionON"(TRUE) -> ()  [unwired: 1 in, 1 out]
                    n223 = local read "TestTime"() -> (w607:dbl)
                    n224 = To Double Precision Float(number=w610) -> (double precision float=w608:dbl)
                    n225 = shared-variable "My Computer\\michelle_library.lvlib\\GlobalTime"() -> (w603:dbl)  [unwired: 1 in, 1 out]
                    n226 = Subtract(x=w608, y=w607) -> (x-y=w611:dbl)
                    n227 = shared-variable "My Computer\\michelle_library.lvlib\\Frame_clock"() -> (w602:u32)  [unwired: 1 in, 1 out]
                    n228 = Build Array(221, w611, w603, w602) -> (w606:T1)
                    n229 = Build Array (concatenate) ("Build Matrix")(w605, w606) -> (w604:T1)
                    n230 = local write "ConsTS"(w604) -> ()
                    "ConsumptionGo" <- TRUE
                  }
                  frame #1 {
                    n231 = Get Date/Time In Seconds() -> (seconds since 1Jan1904=w635:timestamp)
                    n232 = shared-variable "My Computer\\michelle_library.lvlib\\ConsumptionON"(FALSE) -> ()  [unwired: 1 in, 1 out]
                    n233 = local write "ConsumptionGo"(FALSE ("ConsumptionGo")) -> ()
                    n234 = local write "Watch_Display"(FALSE ("Watch_Display")) -> ()
                    n235 = local read "TestTime"() -> (w632:dbl)
                    n236 = To Double Precision Float(number=w635) -> (double precision float=w633:dbl)
                    n237 = shared-variable "My Computer\\michelle_library.lvlib\\GlobalTime"() -> (w628:dbl)  [unwired: 1 in, 1 out]
                    n238 = Subtract(x=w633, y=w632) -> (x-y=w636:dbl)
                    n239 = shared-variable "My Computer\\michelle_library.lvlib\\Frame_clock"() -> (w627:u32)  [unwired: 1 in, 1 out]
                    n240 = Build Array(222, w636, w628, w627) -> (w629:T1)
                    n241 = Build Array (concatenate) ("Build Matrix")(w631, w629) -> (w630:T1)
                    n242 = local write "Its"(0) -> ()
                    n243 = local write "ConsTS"(w630) -> ()
                  }
                }
              }
              frame True {
              }
            }
          }
        }
        n244 = Wait (ms)(milliseconds to wait=u32 5) -> ()  [unwired: 1 out]
        n245 = shared-variable "My Computer\\michelle_library.lvlib\\Stop"() -> (w593:bool)  [unwired: 1 in, 1 out]
      }
      n246 = flat-sequence {
        frame #0 {
          n247 = while {
            stop <- w657 stop-if-true
            n248 = shared-variable "My Computer\\michelle_library.lvlib\\Stim_loaded"() -> (w657:bool)  [unwired: 1 in, 1 out]
            "Stimuli Loaded" <- w657
          }
          n249 = Wait (ms)(milliseconds to wait=u32 10) -> ()  [unwired: 1 out]
        }
        frame #1 {
          n250 = Get Date/Time In Seconds() -> (seconds since 1Jan1904=w663:timestamp)
          n251 = local read "TestTime"() -> (w662:dbl)
          n252 = To Double Precision Float(number=w663) -> (double precision float=w661:dbl)
          n253 = shared-variable "My Computer\\michelle_library.lvlib\\InitiatedLag"() -> (w660:dbl)  [unwired: 1 in, 1 out]
          n254 = Subtract(x=w661, y=w662) -> (x-y=w658:dbl)
          n255 = Subtract(x=w658, y=w660) -> (x-y=→"Lag2":dbl)
        }
        frame #2 {
          n256 = local read "TestTime"() -> (w664:dbl)
          n257 = local read "Lag2"() -> (w665:dbl)
          n258 = Add(x=w664, y=w665) -> (x+y=w666:dbl)
          n259 = local write "TestTime"(w666) -> ()
        }
        frame #3 {
          n260 = shared-variable "My Computer\\michelle_library.lvlib\\Timings"() -> (→"Timings":dbl[])  [unwired: 1 in, 1 out]
          n261 = shared-variable "My Computer\\michelle_library.lvlib\\Stim_ID"() -> (→"Stim_ID":dbl[])  [unwired: 1 in, 1 out]
          n262 = Wait (ms)(milliseconds to wait=u32 10) -> ()  [unwired: 1 out]
          n263 = shared-variable "My Computer\\michelle_library.lvlib\\Reward_mat"() -> (→"Reward_mat":dbl[])  [unwired: 1 in, 1 out]
          n264 = shared-variable "My Computer\\michelle_library.lvlib\\Num_trials"() -> (w670:u32)  [unwired: 1 in, 1 out]
          n265 = Initialize Array(0.0 ("element"), w670) -> (→"Rewarded trials":dbl[])
        }
        frame #4 {
          n266 = while {
            shift-right: [w786] -> _
            shift-left: _ -> [w784]
            shift-right: [w782] -> _
            shift-left: _ -> [w781]
            shift-right: [w776] -> _
            shift-left: _ -> [w774]
            stop <- w787 stop-if-true
            n267 = local read "ConsumptionGo"() -> (w776:bool)
            n268 = shared-variable "My Computer\\michelle_library.lvlib\\Display"() -> (w782:bool)  [unwired: 1 in, 1 out]
            n269 = local read "Time_out"() -> (w786:bool)
            n270 = Wait (ms)(milliseconds to wait=u32 10) -> ()  [unwired: 1 out]
            n271 = Not(x=w786) -> (.not. x?=w785:bool)
            n272 = Not(x=w782) -> (.not. x?=w780:bool)
            n273 = Not(x=w776) -> (.not. x?=w777:bool)
            n274 = And(x=w785, y=w784) -> (x .and. y?=w779:bool)
            n275 = And(x=w781, y=w780) -> (x .and. y?=w775:bool)
            n276 = local read "Time_out"() -> (w783:bool)
            n277 = And(x=w774, y=w777) -> (x .and. y?=w773:bool)
            n278 = Or(x=w779, y=w775) -> (x .or. y?=w772:bool)
            n279 = Or(x=w772, y=w773) -> (x .or. y?=w771:bool)
            n280 = case shown="True" w771 {
              tunnel: w783 -> [w788 _]
              frame False {
                n281 = case shown="False" w788 {
                  frame False {
                    n282 = local read "ISI start time"() -> (w791:dbl)
                    n283 = local read "Time"() -> (w790:dbl)
                    n284 = Subtract(x=w790, y=w791) -> (x-y=w789:dbl)
                    n285 = shared-variable "My Computer\\michelle_library.lvlib\\ISI"(w789) -> ()  [unwired: 1 in, 1 out]
                    n286 = local write "ISI"(w789) -> ()
                  }
                  frame True {
                    n287 = local read "Time"() -> (w796:dbl)
                    n288 = Subtract(x=w796, y=0.11) -> (x-y=w793:dbl)
                    n289 = local write "ISI start time"(w793) -> ()
                    n290 = local read "Time"() -> (w794:dbl)
                    n291 = Subtract(x=w794, y=w793) -> (x-y=w792:dbl)
                    n292 = shared-variable "My Computer\\michelle_library.lvlib\\ISI"(w792) -> ()  [unwired: 1 in, 1 out]
                    n293 = local write "ISI"(w792) -> ()
                  }
                }
              }
              frame True {
                n294 = local read "Time"() -> (w801:dbl)
                n295 = Subtract(x=w801, y=0.11) -> (x-y=w798:dbl)
                "ISI start time" <- w798
                n296 = local read "Time"() -> (w799:dbl)
                n297 = Subtract(x=w799, y=w798) -> (x-y=w797:dbl)
                "ISI" <- w797
                n298 = shared-variable "My Computer\\michelle_library.lvlib\\ISI"(w797) -> ()  [unwired: 1 in, 1 out]
              }
            }
            n299 = local read "Stop"() -> (w787:bool)
          }
          n300 = while {
            stop <- w676 stop-if-true
            n301 = local read "Active Trial"() -> (w675:bool)
            n302 = case shown="True" w675 {
              frame False {
              }
              frame True {
                n303 = local write "Time_out"(FALSE) -> ()
                n304 = shared-variable "My Computer\\michelle_library.lvlib\\Timeout"(FALSE) -> ()  [unwired: 1 in, 1 out]
              }
            }
            n305 = Wait (ms)(milliseconds to wait=5) -> ()  [unwired: 1 out]
            n306 = shared-variable "My Computer\\michelle_library.lvlib\\Stop"() -> (w676:bool)  [unwired: 1 in, 1 out]
          }
          n307 = while {
            stop <- w697 stop-if-true
            n308 = shared-variable "My Computer\\michelle_library.lvlib\\Trial"() -> (w687:u32)  [unwired: 1 in, 1 out]
            n309 = Wait (ms)(milliseconds to wait=u32 10) -> ()  [unwired: 1 out]
            n310 = local read "Timings"() -> (w689:dbl[])
            n311 = local read "Time since lick"() -> (w696:dbl)
            n312 = Decrement(x=w687) -> (x-1=w686:u32)
            n313 = Index Array(array=w689, index=w686) -> (element=w688:dbl)
            n314 = Less?(x=w696, y=w688) -> (x < y?=w695:bool)
            n315 = shared-variable "My Computer\\michelle_library.lvlib\\Display"() -> (w692:bool)  [unwired: 1 in, 1 out]
            n316 = local read "ConsumptionGo"() -> (w684:bool)
            n317 = local read "Lick"() -> (w694:bool)
            n318 = And(x=w694, y=w695) -> (x .and. y?=w690:bool)
            n319 = Not(x=w692) -> (.not. x?=w691:bool)
            n320 = local read "Active Trial"() -> (w679:bool)
            n321 = And(x=w691, y=w690) -> (x .and. y?=w683:bool)
            n322 = Not(x=w684) -> (.not. x?=w685:bool)
            n323 = And(x=w683, y=w685) -> (x .and. y?=w681:bool)
            n324 = Not(x=w679) -> (.not. x?=w682:bool)
            n325 = And(x=w681, y=w682) -> (x .and. y?=w680:bool)
            n326 = case shown="True" w680 {
              frame False {
              }
              frame True {
                n327 = flat-sequence {
                  frame #0 {
                    w698 = TRUE
                    n328 = local read "TimeOutDuration"() -> (w699:i32)
                    n329 = xnode "DisplayOn 3"("C/DIO3 (DIO3)"=w698) -> ()  [unwired: 1 in, 1 out]
                    n330 = shared-variable "My Computer\\michelle_library.lvlib\\Timeout"(w698) -> ()  [unwired: 1 in, 1 out]
                    n331 = Wait (ms)(milliseconds to wait=w699) -> ()  [unwired: 1 out]
                    "Time_out" <- w698
                  }
                  frame #1 {
                    w735 = FALSE ("Timeout")
                    n332 = xnode "DisplayOn 4"("C/DIO3 (DIO3)"=w735) -> ()  [unwired: 1 in, 1 out]
                    n333 = local write "Time_out"(w735) -> ()
                    n334 = shared-variable "My Computer\\michelle_library.lvlib\\Timeout"(w735) -> ()  [unwired: 1 in, 1 out]
                  }
                }
              }
            }
            n335 = local read "Stop"() -> (w697:bool)
          }
          n336 = while {
            shift-right: [w848] -> _
            shift-left: _ -> [w847]
            shift-right: [w840] -> _
            shift-left: _ -> [w841]
            stop <- w850 stop-if-true
            n337 = local read "Active Trial"() -> (w845:bool)
            n338 = Wait (ms)(milliseconds to wait=u32 10) -> ()  [unwired: 1 out]
            n339 = local read "Lick"() -> (w846:bool)
            n340 = And(x=w845, y=w846) -> (x .and. y?=w844:bool)
            n341 = Or(x="Give reward", y=w844) -> (x .or. y?=w843:bool)
            n342 = case shown="True" w843 {
              tunnel: [w852 w859] -> w848
              tunnel: w847 -> [w852 w858]
              tunnel: w841 -> [w851 w856]
              tunnel: [w851 w855] -> w840
              frame False {
              }
              frame True {
                n343 = flat-sequence {
                  tunnel: w856 -> [w865]
                  tunnel: [w862] -> w853
                  tunnel: [w921] -> w854
                  tunnel: w853 -> [w919]
                  tunnel: [w965] -> w855
                  tunnel: w854 -> [w965]
                  frame #0 {
                    w880 = TRUE ("C/DIO0 (DIO0)")
                    n344 = Get Date/Time In Seconds() -> (seconds since 1Jan1904=w869:timestamp)
                    n345 = local write "Time_out"(FALSE) -> ()
                    n346 = shared-variable "My Computer\\michelle_library.lvlib\\Timeout"(FALSE) -> ()  [unwired: 1 in, 1 out]
                    n347 = local write "GoAhead"(FALSE) -> ()
                    n348 = Wait (ms)(milliseconds to wait=u32 100) -> ()  [unwired: 1 out]
                    n349 = local read "TestTime"() -> (w863:dbl)
                    n350 = shared-variable "My Computer\\michelle_library.lvlib\\Trial"() -> (w879:u32)  [unwired: 1 in, 1 out]
                    n351 = shared-variable "My Computer\\michelle_library.lvlib\\GlobalReward"() -> (w871:dbl)  [unwired: 1 in, 1 out]
                    n352 = To Double Precision Float(number=w869) -> (double precision float=w868:dbl)
                    n353 = shared-variable "My Computer\\michelle_library.lvlib\\GlobalTime"() -> (w861:dbl)  [unwired: 1 in, 1 out]
                    n354 = local read "Rewarded trials"() -> (w877:dbl[])
                    n355 = Subtract(x=w868, y=w863) -> (x-y=w867:dbl)
                    n356 = xnode "Reward 3"("C/DIO0 (DIO0)"=w880) -> ()  [unwired: 1 in, 1 out]
                    n357 = Decrement(x=w879) -> (x-1=w878:u32)
                    n358 = shared-variable "My Computer\\michelle_library.lvlib\\Frame_clock"() -> (w860:u32)  [unwired: 1 in, 1 out]
                    n359 = Increment(x=w871) -> (x+1=w870:dbl)
                    n360 = Replace Array Subset(array=w877, new element=1.0 ("new element/subarray"), index=w878) -> (w875:dbl[])
                    n361 = Build Array(551, w867, w861, w860) -> (w866:T1)
                    n362 = local write "Rewarded trials"(w875) -> ()
                    n363 = shared-variable "My Computer\\michelle_library.lvlib\\GlobalReward"(w870) -> ()  [unwired: 1 in, 1 out]
                    n364 = Build Array (concatenate) ("Build Matrix")(w865, w866) -> (w862:T1)
                    n365 = local write "RewTS"(w862) -> ()
                    "Reward" <- w880
                    "Watch_Display" <- w880
                  }
                  frame #1 {
                    w929 = FALSE ("C/DIO0 (DIO0)")
                    n366 = Get Date/Time In Seconds() -> (seconds since 1Jan1904=w926:timestamp)
                    n367 = local read "TestTime"() -> (w920:dbl)
                    n368 = local write "Give reward"(FALSE ("Give reward")) -> ()
                    n369 = Wait (ms)(milliseconds to wait=u32 20) -> ()  [unwired: 1 out]
                    n370 = shared-variable "My Computer\\michelle_library.lvlib\\GlobalTime"() -> (w918:dbl)  [unwired: 1 in, 1 out]
                    n371 = To Double Precision Float(number=w926) -> (double precision float=w925:dbl)
                    n372 = xnode "Reward 4"("C/DIO0 (DIO0)"=w929) -> ()  [unwired: 1 in, 1 out]
                    n373 = local write "Reward"(w929) -> ()
                    n374 = Subtract(x=w925, y=w920) -> (x-y=w924:dbl)
                    n375 = shared-variable "My Computer\\michelle_library.lvlib\\Frame_clock"() -> (w917:u32)  [unwired: 1 in, 1 out]
                    n376 = Build Array(552, w924, w918, w917) -> (w922:T1)
                    n377 = Build Array (concatenate) ("Build Matrix")(w919, w922) -> (w921:T1)
                    n378 = local write "RewTS"(w921) -> ()
                  }
                  frame #2 {
                    n379 = Wait (ms)(milliseconds to wait=u32 50) -> ()  [unwired: 1 out]
                  }
                }
                n380 = Increment(x=w858) -> (x+1=w859:u16)
                "Rewards" <- w859
                n381 = local write "Active Trial"(FALSE ("Active Trial")) -> ()
              }
            }
            n382 = local read "Stop"() -> (w850:bool)
          }
          n383 = while {
            stop <- w815 stop-if-true
            n384 = shared-variable "My Computer\\michelle_library.lvlib\\Trial"() -> (w811:u32)  [unwired: 1 in, 1 out]
            n385 = shared-variable "My Computer\\michelle_library.lvlib\\Trial"() -> (w807:u32)  [unwired: 1 in, 1 out]
            n386 = Wait (ms)(milliseconds to wait=u32 10) -> ()  [unwired: 1 out]
            n387 = local read "Rewarded trials"() -> (w808:dbl[])
            n388 = local read "Reward_mat"() -> (w810:dbl[])
            n389 = Decrement(x=w811) -> (x-1=w812:u32)
            n390 = Decrement(x=w807) -> (x-1=w806:u32)
            n391 = Index Array(array=w810, index=w812) -> (element=w813:dbl)
            n392 = Index Array(array=w808, index=w806) -> (element=w805:dbl)
            n393 = Equal To 0?(x=w805) -> (x = 0?=w804:bool)
            n394 = Equal?(x=w813, y=1.0) -> (x = y?=w803:bool)
            n395 = And(x=w803, y=w804) -> (x .and. y?=w802:bool)
            n396 = case shown="True" w802 {
              frame False {
                n397 = local write "Active Trial"(FALSE ("Active_trial")) -> ()
              }
              frame True {
                n398 = shared-variable "My Computer\\michelle_library.lvlib\\Trial"() -> (w818:u32)  [unwired: 1 in, 1 out]
                n399 = local read "Stim_ID"() -> (w820:dbl[])
                n400 = Decrement(x=w818) -> (x-1=w819:u32)
                n401 = Index Array(array=w820, index=w819) -> (element=w817:dbl)
                n402 = case shown="1, Default" w817 {
                  frame 1, Default {
                    n403 = shared-variable "My Computer\\michelle_library.lvlib\\ISI_Time"() -> (w826:dbl)  [unwired: 1 in, 1 out]
                    n404 = local read "ActiveTime"() -> (w821:dbl)
                    n405 = Less?(x=w826, y=w821) -> (x < y?=w824:bool)
                    n406 = Greater?(x=w826, y=0.1) -> (0:w823:bool)
                    n407 = And(x=w824, y=w823) -> (x .and. y?=w822:bool)
                    n408 = case shown="True" w822 {
                      frame False {
                        n409 = local write "Active Trial"(FALSE ("Active Trial")) -> ()
                      }
                      frame True {
                        n410 = local read "Time"() -> (w830:dbl)
                        n411 = local write "Active Trial"(TRUE ("Active Trial")) -> ()
                        n412 = Add(x=w830, y=-0.11) -> (x+y=w828:dbl)
                        n413 = local write "Time of last lick"(w828) -> ()
                      }
                    }
                  }
                  frame 2 {
                    n414 = shared-variable "My Computer\\michelle_library.lvlib\\ISI_Time"() -> (w836:dbl)  [unwired: 1 in, 1 out]
                    n415 = local read "ActiveTime"() -> (w832:dbl)
                    n416 = Less?(x=w836, y=w832) -> (x < y?=w834:bool)
                    n417 = Greater?(x=w836, y=0.1) -> (0:w835:bool)
                    n418 = And(x=w835, y=w834) -> (x .and. y?=w833:bool)
                    n419 = case shown="True" w833 {
                      frame False {
                        n420 = local write "Active Trial"(FALSE ("Active Trial")) -> ()
                      }
                      frame True {
                        "Active Trial" <- TRUE ("Active Trial")
                      }
                    }
                  }
                }
              }
            }
            n421 = local read "Stop"() -> (w815:bool)
          }
        }
      }
      n422 = flat-sequence {
        frame #0 {
          n423 = xnode "Encoder 4"("Reset Counter"=TRUE) -> ()  [unwired: 1 in, 4 out]
        }
        frame #1 {
          n424 = while {
            stop <- w388 stop-if-true
            n425 = xnode "Encoder 3"() -> ("Counter Value"=w390:i32)  [unwired: 2 in, 3 out]
            n426 = Multiply(x=w390, y=-1) -> (x*y=w387:i32)
            "VidFrameClock" <- w387
            n427 = Equal?(x=w387, y=720000) -> (x = y?=w388:bool)
            n428 = shared-variable "My Computer\\michelle_library.lvlib\\VidFrameClock1"(w387) -> ()  [unwired: 1 in, 1 out]
            n429 = local write "Stop"(w388) -> ()
            n430 = Wait (ms)(milliseconds to wait=u32 1) -> ()  [unwired: 1 out]
          }
        }
        frame #2 {
          n431 = local read "Stop"() -> (w438:bool)
          n432 = shared-variable "My Computer\\michelle_library.lvlib\\Stop"(w438) -> ()  [unwired: 1 in, 1 out]
        }
      }
    }
  }
